vi "Calculate I2C API.vi"(8 "error in (no error)":errorcluster, 11 "Devices DVR In":refnum<data-value>) -> (0 "error out":errorcluster, 3 "Devices DVR Out":refnum<data-value>)   [LabVIEW 2020, in "Devices.lvclass"]
uses:
  Devices.lvclass
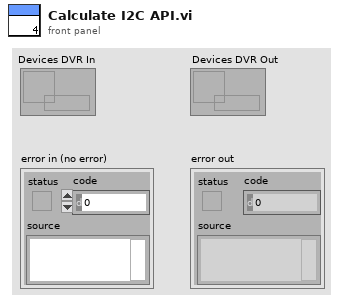
[diagram p1: front panel]
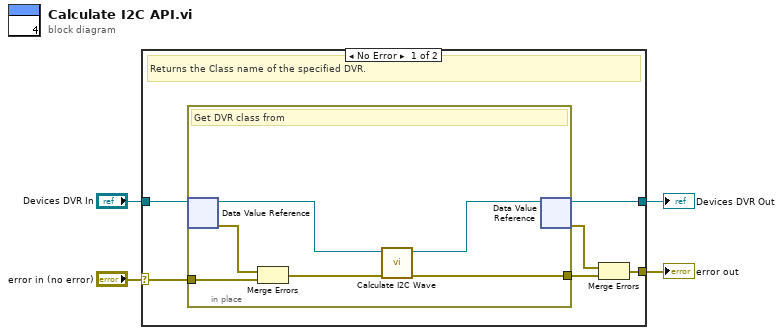
[diagram p0: block diagram]
diagram:
  n1 = case shown="No Error" "error in (no error)" {
    selector: "error in (no error)" -> [w9 w18]
    tunnel: [w10 w17] -> w1
    tunnel: [w7 w18] -> w3
    tunnel: "Devices DVR In" -> [w5 w17]
    frame No Error {
      # "Returns the Class name of the specified DVR."
      n2 = in-place {
        in-place-border: w9 -> [w16]
        in-place-border: [w13] -> w6
        # "Get DVR class from"
        n3 = in-place-dvr #1(w5) -> (w11:refnum<class "Devices.lvclass">, w15:errorcluster)
        n4 = Merge Errors(w15, w16) -> (w14:errorcluster)
        n5 = call-dynamic "Calculate I2C Wave.vi"("error in (no error)"=w14, "Devices in"=w11) -> ("error out"=w13:errorcluster, "Devices out"=w12:refnum<class "Devices.lvclass">)  [unwired: 8 in]
        n6 = in-place-dvr #1(w12) -> (w10:refnum<data-value>, w8:errorcluster)
      }
      n7 = Merge Errors(w8, w6) -> (w7:errorcluster)
    }
    frame Error {
    }
  }
  "error out" <- w3
  "Devices DVR Out" <- w1
